vi "WriteForceIni1#.vi"(1 "configuration file path":path=path "E:/LabVIEW/福尔达/AppData") -> ()   [LabVIEW 2018]
uses:
  <vilib>/Utility/config.llb/Write Key (Double).vi
  <vilib>/Utility/config.llb/NI_LVConfig.lvlib
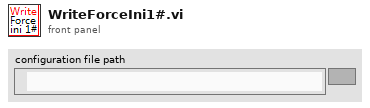
[diagram p1: front panel]
types:
  T1 = typedef "NI_LVConfig.lvlib/Config Data RefNum.ctl" = refnum<k1>
  T2 = cluster{"选择":enum16{"Fx", "Fy", "Fz", "Mx", "My", "Mz"}, "系数x":sgl, "系数+":sgl, "上限":sgl, "下限":sgl, "Ymax":dbl, "Ymin":dbl, "点数":dbl, "锁系数x":sgl, "锁上限":sgl, "锁下限":sgl, "锁系数+":sgl, "起点":dbl, "终点":dbl, "锁起点":dbl, "锁终点":dbl, "上参考":sgl, "下参考":sgl, "基准":sgl}
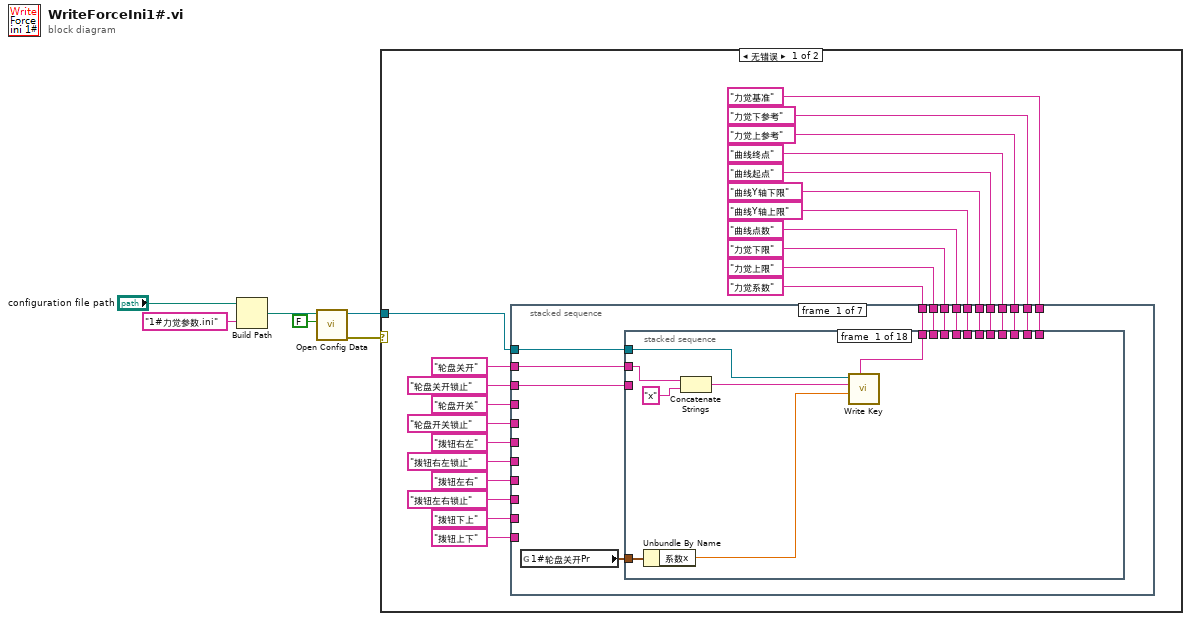
[diagram p0: block diagram]
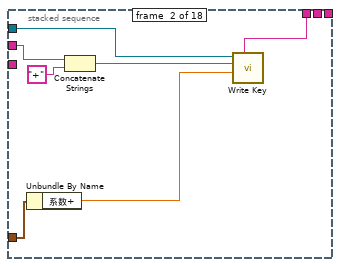
[diagram p2: hidden frame]
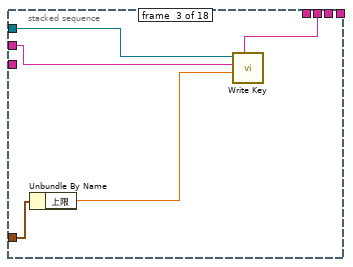
[diagram p3: hidden frame]
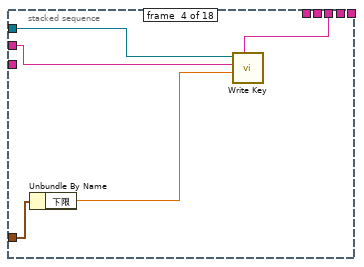
[diagram p4: hidden frame]
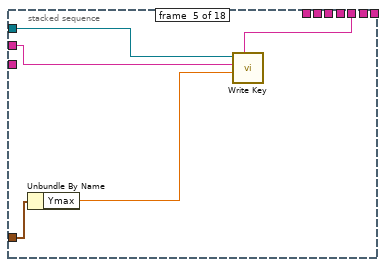
[diagram p5: hidden frame]
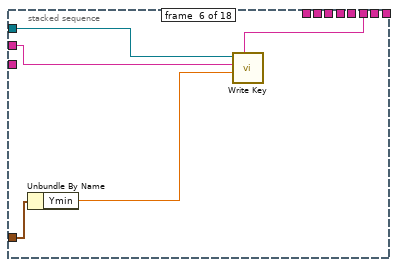
[diagram p6: hidden frame]
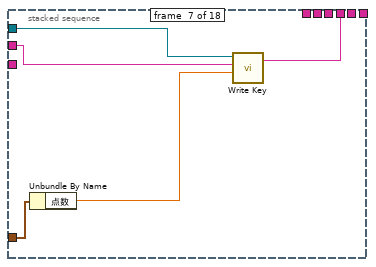
[diagram p7: hidden frame]
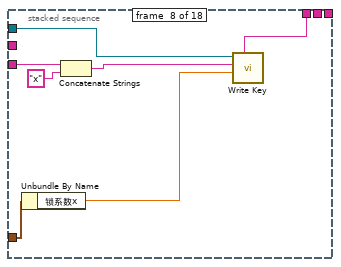
[diagram p8: hidden frame]
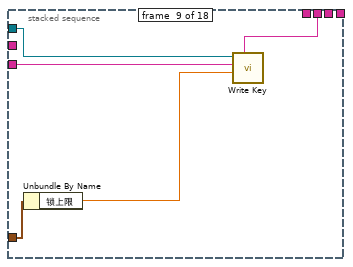
[diagram p9: hidden frame]
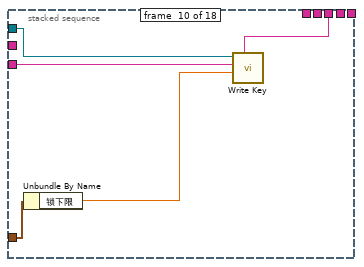
[diagram p10: hidden frame]
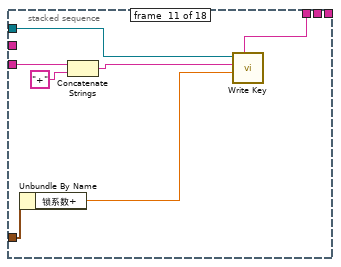
[diagram p11: hidden frame]
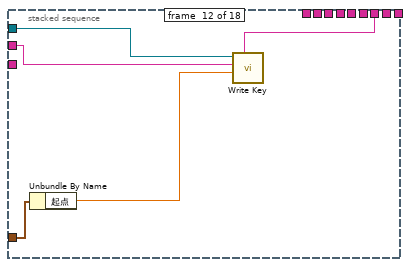
[diagram p12: hidden frame]
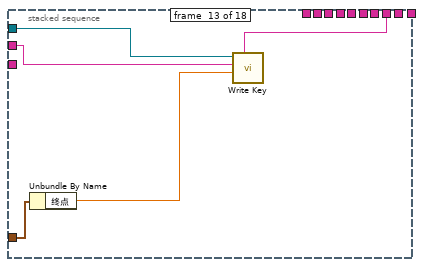
[diagram p13: hidden frame]
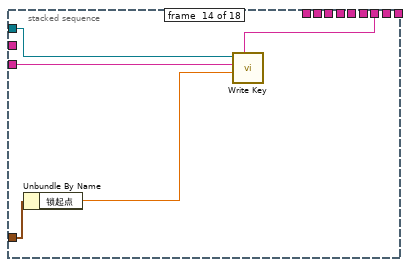
[diagram p14: hidden frame]
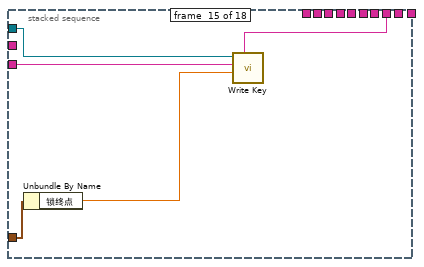
[diagram p15: hidden frame]
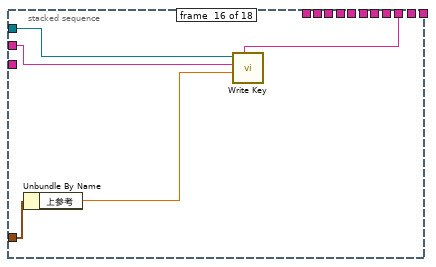
[diagram p16: hidden frame]
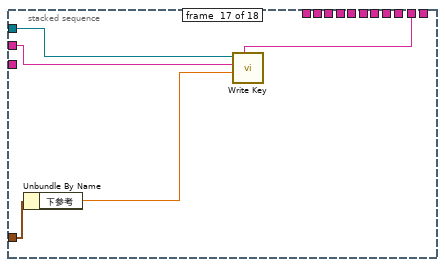
[diagram p17: hidden frame]
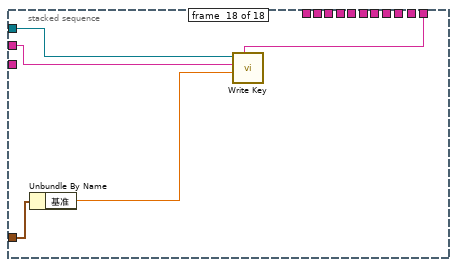
[diagram p18: hidden frame]
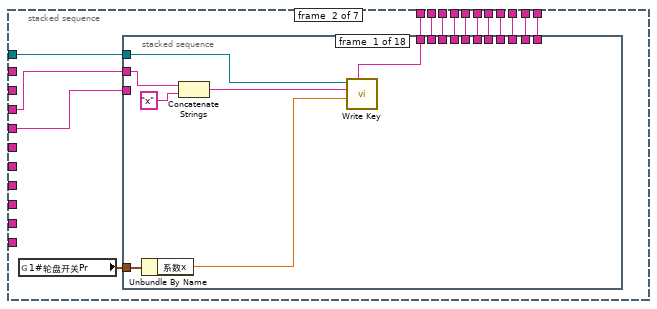
[diagram p19: hidden frame]
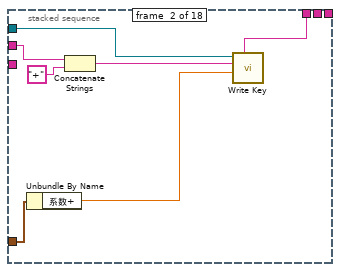
[diagram p20: hidden frame]
diagram:
  n1 = Build Path(base path="configuration file path", name or relative path="1#力觉参数.ini" ("名称或相对路径")) -> (appended path=w6:path)
  n2 = call <vilib>:"Open Config Data.vi"("create file if necessary (T)"=FALSE, "configuration file path"=w6) -> ("error out"=w1:errorcluster, "refnum"=w4:T1)  [unwired: 7 in, 1 out]
  n3 = case shown="无错误" w1 {
    tunnel: w4 -> [w12 w639]
    frame No Error {
      n4 = stacked-sequence {
        tunnel: w12 -> [w32 w147 w260 w373 w485 w563 w637]
        tunnel: "轮盘关开" -> [w42 _ _ _ _ _ _]
        tunnel: "拨钮上下" -> [_ _ _ _ _ w559 _]
        tunnel: "拨钮下上" -> [_ _ _ _ w481 _ _]
        tunnel: "拨钮左右" -> [_ _ _ w369 _ _ _]
        tunnel: "拨钮右左" -> [_ _ w256 _ _ _ _]
        tunnel: "轮盘开关锁止" -> [_ w142 _ _ _ _ _]
        tunnel: "轮盘开关" -> [_ w143 _ _ _ _ _]
        tunnel: "轮盘关开锁止" -> [w33 _ _ _ _ _ _]
        tunnel: "力觉系数" -> [w41 w155 w268 w381 w493 w571 _]
        tunnel: "力觉上限" -> [w40 w154 w267 w380 w492 w570 _]
        tunnel: "力觉下限" -> [w39 w153 w266 w379 w491 w569 _]
        tunnel: "曲线点数" -> [w38 w152 w265 w378 w490 w568 _]
        tunnel: "曲线Y轴上限" -> [w37 w151 w264 w377 w489 w567 _]
        tunnel: "曲线Y轴下限" -> [w36 w150 w263 w376 w488 w566 _]
        tunnel: "曲线起点" -> [w35 w149 w262 w375 w487 w565 _]
        tunnel: "曲线终点" -> [w34 w148 w261 w374 w486 w564 _]
        tunnel: "力觉上参考" -> [w31 w146 w259 w372 w484 w562 _]
        tunnel: "力觉下参考" -> [w30 w145 w258 w371 w483 w561 _]
        tunnel: "力觉基准" -> [w29 w144 w257 w370 w482 w560 _]
        tunnel: "拨钮右左锁止" -> [_ _ w255 _ _ _ _]
        tunnel: "拨钮左右锁止" -> [_ _ _ w368 _ _ _]
        frame #0 {
          n5 = global read "全局F参数.vi" "1#轮盘关开Pr"() -> (w43:T2)
          n6 = stacked-sequence {
            tunnel: w42 -> [w44 w51 w59 w64 w69 w74 w79 _ _ _ _ w108 w113 _ _ w127 w132 w137]
            tunnel: w43 -> [w50 w57 w62 w67 w72 w77 w82 w89 w94 w99 w106 w111 w116 w121 w126 w131 w136 w141]
            tunnel: w32 -> [w48 w55 w60 w65 w70 w75 w80 w87 w92 w97 w104 w109 w114 w119 w124 w129 w134 w139]
            tunnel: w41 -> [w47 w54 _ _ _ _ _ w86 _ _ w100 _ _ _ _ _ _ _]
            tunnel: w40 -> [_ _ w58 _ _ _ _ _ w90 _ _ _ _ _ _ _ _ _]
            tunnel: w39 -> [_ _ _ w63 _ _ _ _ _ w95 _ _ _ _ _ _ _ _]
            tunnel: w38 -> [_ _ _ _ _ _ w78 _ _ _ _ _ _ _ _ _ _ _]
            tunnel: w37 -> [_ _ _ _ w68 _ _ _ _ _ _ _ _ _ _ _ _ _]
            tunnel: w36 -> [_ _ _ _ _ w73 _ _ _ _ _ _ _ _ _ _ _ _]
            tunnel: w35 -> [_ _ _ _ _ _ _ _ _ _ _ w107 _ w117 _ _ _ _]
            tunnel: w34 -> [_ _ _ _ _ _ _ _ _ _ _ _ w112 _ w122 _ _ _]
            tunnel: w33 -> [_ _ _ _ _ _ _ w85 w91 w96 w103 _ _ w118 w123 _ _ _]
            tunnel: w31 -> [_ _ _ _ _ _ _ _ _ _ _ _ _ _ _ w128 _ _]
            tunnel: w30 -> [_ _ _ _ _ _ _ _ _ _ _ _ _ _ _ _ w133 _]
            tunnel: w29 -> [_ _ _ _ _ _ _ _ _ _ _ _ _ _ _ _ _ w138]
            frame #0 {
              n7 = Unbundle By Name(w50) -> ("系数x"=w49:sgl)
              n8 = Concatenate Strings(w44, "x") -> (w45:string)
              n9 = call-poly <vilib>:"Write Key.vi"("section"=w47, "value"=w49, "key"=w45, "refnum"=w48) -> ()  [unwired: 5 in, 3 out]
            }
            frame #1 {
              n10 = Unbundle By Name(w57) -> ("系数+"=w56:sgl)
              n11 = Concatenate Strings(w51, "+") -> (w52:string)
              n12 = call-poly <vilib>:"Write Key.vi"("section"=w54, "value"=w56, "key"=w52, "refnum"=w55) -> ()  [unwired: 5 in, 3 out]
            }
            frame #2 {
              n13 = Unbundle By Name(w62) -> ("上限"=w61:sgl)
              n14 = call-poly <vilib>:"Write Key.vi"("section"=w58, "value"=w61, "key"=w59, "refnum"=w60) -> ()  [unwired: 5 in, 3 out]
            }
            frame #3 {
              n15 = Unbundle By Name(w67) -> ("下限"=w66:sgl)
              n16 = call-poly <vilib>:"Write Key.vi"("section"=w63, "value"=w66, "key"=w64, "refnum"=w65) -> ()  [unwired: 5 in, 3 out]
            }
            frame #4 {
              n17 = Unbundle By Name(w72) -> ("Ymax"=w71:dbl)
              n18 = call-poly <vilib>:"Write Key.vi"("section"=w68, "value"=w71, "key"=w69, "refnum"=w70) -> ()  [unwired: 5 in, 3 out]
            }
            frame #5 {
              n19 = Unbundle By Name(w77) -> ("Ymin"=w76:dbl)
              n20 = call-poly <vilib>:"Write Key.vi"("section"=w73, "value"=w76, "key"=w74, "refnum"=w75) -> ()  [unwired: 5 in, 3 out]
            }
            frame #6 {
              n21 = Unbundle By Name(w82) -> ("点数"=w81:dbl)
              n22 = call-poly <vilib>:"Write Key.vi"("section"=w78, "value"=w81, "key"=w79, "refnum"=w80) -> ()  [unwired: 5 in, 3 out]
            }
            frame #7 {
              n23 = Unbundle By Name(w89) -> ("锁系数x"=w88:sgl)
              n24 = Concatenate Strings(w85, "x") -> (w84:string)
              n25 = call-poly <vilib>:"Write Key.vi"("section"=w86, "value"=w88, "key"=w84, "refnum"=w87) -> ()  [unwired: 5 in, 3 out]
            }
            frame #8 {
              n26 = Unbundle By Name(w94) -> ("锁上限"=w93:sgl)
              n27 = call-poly <vilib>:"Write Key.vi"("section"=w90, "value"=w93, "key"=w91, "refnum"=w92) -> ()  [unwired: 5 in, 3 out]
            }
            frame #9 {
              n28 = Unbundle By Name(w99) -> ("锁下限"=w98:sgl)
              n29 = call-poly <vilib>:"Write Key.vi"("section"=w95, "value"=w98, "key"=w96, "refnum"=w97) -> ()  [unwired: 5 in, 3 out]
            }
            frame #10 {
              n30 = Unbundle By Name(w106) -> ("锁系数+"=w105:sgl)
              n31 = Concatenate Strings(w103, "+") -> (w102:string)
              n32 = call-poly <vilib>:"Write Key.vi"("section"=w100, "value"=w105, "key"=w102, "refnum"=w104) -> ()  [unwired: 5 in, 3 out]
            }
            frame #11 {
              n33 = Unbundle By Name(w111) -> ("起点"=w110:dbl)
              n34 = call-poly <vilib>:"Write Key.vi"("section"=w107, "value"=w110, "key"=w108, "refnum"=w109) -> ()  [unwired: 5 in, 3 out]
            }
            frame #12 {
              n35 = Unbundle By Name(w116) -> ("终点"=w115:dbl)
              n36 = call-poly <vilib>:"Write Key.vi"("section"=w112, "value"=w115, "key"=w113, "refnum"=w114) -> ()  [unwired: 5 in, 3 out]
            }
            frame #13 {
              n37 = Unbundle By Name(w121) -> ("锁起点"=w120:dbl)
              n38 = call-poly <vilib>:"Write Key.vi"("section"=w117, "value"=w120, "key"=w118, "refnum"=w119) -> ()  [unwired: 5 in, 3 out]
            }
            frame #14 {
              n39 = Unbundle By Name(w126) -> ("锁终点"=w125:dbl)
              n40 = call-poly <vilib>:"Write Key.vi"("section"=w122, "value"=w125, "key"=w123, "refnum"=w124) -> ()  [unwired: 5 in, 3 out]
            }
            frame #15 {
              n41 = Unbundle By Name(w131) -> ("上参考"=w130:sgl)
              n42 = call-poly <vilib>:"Write Key.vi"("section"=w128, "value"=w130, "key"=w127, "refnum"=w129) -> ()  [unwired: 5 in, 3 out]
            }
            frame #16 {
              n43 = Unbundle By Name(w136) -> ("下参考"=w135:sgl)
              n44 = call-poly <vilib>:"Write Key.vi"("section"=w133, "value"=w135, "key"=w132, "refnum"=w134) -> ()  [unwired: 5 in, 3 out]
            }
            frame #17 {
              n45 = Unbundle By Name(w141) -> ("基准"=w140:sgl)
              n46 = call-poly <vilib>:"Write Key.vi"("section"=w138, "value"=w140, "key"=w137, "refnum"=w139) -> ()  [unwired: 5 in, 3 out]
            }
          }
        }
        frame #1 {
          n47 = global read "全局F参数.vi" "1#轮盘开关Pr"() -> (w156:T2)
          n48 = stacked-sequence {
            tunnel: w143 -> [w157 w164 w172 w177 w182 w187 w192 _ _ _ _ w221 w226 _ _ w240 w245 w250]
            tunnel: w156 -> [w163 w170 w175 w180 w185 w190 w195 w202 w207 w212 w219 w224 w229 w234 w239 w244 w249 w254]
            tunnel: w147 -> [w161 w168 w173 w178 w183 w188 w193 w200 w205 w210 w217 w222 w227 w232 w237 w242 w247 w252]
            tunnel: w155 -> [w160 w167 _ _ _ _ _ w199 _ _ w213 _ _ _ _ _ _ _]
            tunnel: w154 -> [_ _ w171 _ _ _ _ _ w203 _ _ _ _ _ _ _ _ _]
            tunnel: w153 -> [_ _ _ w176 _ _ _ _ _ w208 _ _ _ _ _ _ _ _]
            tunnel: w152 -> [_ _ _ _ _ _ w191 _ _ _ _ _ _ _ _ _ _ _]
            tunnel: w151 -> [_ _ _ _ w181 _ _ _ _ _ _ _ _ _ _ _ _ _]
            tunnel: w150 -> [_ _ _ _ _ w186 _ _ _ _ _ _ _ _ _ _ _ _]
            tunnel: w149 -> [_ _ _ _ _ _ _ _ _ _ _ w220 _ w230 _ _ _ _]
            tunnel: w148 -> [_ _ _ _ _ _ _ _ _ _ _ _ w225 _ w235 _ _ _]
            tunnel: w142 -> [_ _ _ _ _ _ _ w198 w204 w209 w216 _ _ w231 w236 _ _ _]
            tunnel: w146 -> [_ _ _ _ _ _ _ _ _ _ _ _ _ _ _ w241 _ _]
            tunnel: w145 -> [_ _ _ _ _ _ _ _ _ _ _ _ _ _ _ _ w246 _]
            tunnel: w144 -> [_ _ _ _ _ _ _ _ _ _ _ _ _ _ _ _ _ w251]
            frame #0 {
              n49 = Unbundle By Name(w163) -> ("系数x"=w162:sgl)
              n50 = Concatenate Strings(w157, "x") -> (w158:string)
              n51 = call-poly <vilib>:"Write Key.vi"("section"=w160, "value"=w162, "key"=w158, "refnum"=w161) -> ()  [unwired: 5 in, 3 out]
            }
            frame #1 {
              n52 = Unbundle By Name(w170) -> ("系数+"=w169:sgl)
              n53 = Concatenate Strings(w164, "+") -> (w165:string)
              n54 = call-poly <vilib>:"Write Key.vi"("section"=w167, "value"=w169, "key"=w165, "refnum"=w168) -> ()  [unwired: 5 in, 3 out]
            }
            frame #2 {
              n55 = Unbundle By Name(w175) -> ("上限"=w174:sgl)
              n56 = call-poly <vilib>:"Write Key.vi"("section"=w171, "value"=w174, "key"=w172, "refnum"=w173) -> ()  [unwired: 5 in, 3 out]
            }
            frame #3 {
              n57 = Unbundle By Name(w180) -> ("下限"=w179:sgl)
              n58 = call-poly <vilib>:"Write Key.vi"("section"=w176, "value"=w179, "key"=w177, "refnum"=w178) -> ()  [unwired: 5 in, 3 out]
            }
            frame #4 {
              n59 = Unbundle By Name(w185) -> ("Ymax"=w184:dbl)
              n60 = call-poly <vilib>:"Write Key.vi"("section"=w181, "value"=w184, "key"=w182, "refnum"=w183) -> ()  [unwired: 5 in, 3 out]
            }
            frame #5 {
              n61 = Unbundle By Name(w190) -> ("Ymin"=w189:dbl)
              n62 = call-poly <vilib>:"Write Key.vi"("section"=w186, "value"=w189, "key"=w187, "refnum"=w188) -> ()  [unwired: 5 in, 3 out]
            }
            frame #6 {
              n63 = Unbundle By Name(w195) -> ("点数"=w194:dbl)
              n64 = call-poly <vilib>:"Write Key.vi"("section"=w191, "value"=w194, "key"=w192, "refnum"=w193) -> ()  [unwired: 5 in, 3 out]
            }
            frame #7 {
              n65 = Unbundle By Name(w202) -> ("锁系数x"=w201:sgl)
              n66 = Concatenate Strings(w198, "x") -> (w197:string)
              n67 = call-poly <vilib>:"Write Key.vi"("section"=w199, "value"=w201, "key"=w197, "refnum"=w200) -> ()  [unwired: 5 in, 3 out]
            }
            frame #8 {
              n68 = Unbundle By Name(w207) -> ("锁上限"=w206:sgl)
              n69 = call-poly <vilib>:"Write Key.vi"("section"=w203, "value"=w206, "key"=w204, "refnum"=w205) -> ()  [unwired: 5 in, 3 out]
            }
            frame #9 {
              n70 = Unbundle By Name(w212) -> ("锁下限"=w211:sgl)
              n71 = call-poly <vilib>:"Write Key.vi"("section"=w208, "value"=w211, "key"=w209, "refnum"=w210) -> ()  [unwired: 5 in, 3 out]
            }
            frame #10 {
              n72 = Unbundle By Name(w219) -> ("锁系数+"=w218:sgl)
              n73 = Concatenate Strings(w216, "+") -> (w215:string)
              n74 = call-poly <vilib>:"Write Key.vi"("section"=w213, "value"=w218, "key"=w215, "refnum"=w217) -> ()  [unwired: 5 in, 3 out]
            }
            frame #11 {
              n75 = Unbundle By Name(w224) -> ("起点"=w223:dbl)
              n76 = call-poly <vilib>:"Write Key.vi"("section"=w220, "value"=w223, "key"=w221, "refnum"=w222) -> ()  [unwired: 5 in, 3 out]
            }
            frame #12 {
              n77 = Unbundle By Name(w229) -> ("终点"=w228:dbl)
              n78 = call-poly <vilib>:"Write Key.vi"("section"=w225, "value"=w228, "key"=w226, "refnum"=w227) -> ()  [unwired: 5 in, 3 out]
            }
            frame #13 {
              n79 = Unbundle By Name(w234) -> ("锁起点"=w233:dbl)
              n80 = call-poly <vilib>:"Write Key.vi"("section"=w230, "value"=w233, "key"=w231, "refnum"=w232) -> ()  [unwired: 5 in, 3 out]
            }
            frame #14 {
              n81 = Unbundle By Name(w239) -> ("锁终点"=w238:dbl)
              n82 = call-poly <vilib>:"Write Key.vi"("section"=w235, "value"=w238, "key"=w236, "refnum"=w237) -> ()  [unwired: 5 in, 3 out]
            }
            frame #15 {
              n83 = Unbundle By Name(w244) -> ("上参考"=w243:sgl)
              n84 = call-poly <vilib>:"Write Key.vi"("section"=w241, "value"=w243, "key"=w240, "refnum"=w242) -> ()  [unwired: 5 in, 3 out]
            }
            frame #16 {
              n85 = Unbundle By Name(w249) -> ("下参考"=w248:sgl)
              n86 = call-poly <vilib>:"Write Key.vi"("section"=w246, "value"=w248, "key"=w245, "refnum"=w247) -> ()  [unwired: 5 in, 3 out]
            }
            frame #17 {
              n87 = Unbundle By Name(w254) -> ("基准"=w253:sgl)
              n88 = call-poly <vilib>:"Write Key.vi"("section"=w251, "value"=w253, "key"=w250, "refnum"=w252) -> ()  [unwired: 5 in, 3 out]
            }
          }
        }
        frame #2 {
          n89 = global read "全局F参数.vi" "1#拨钮右左Pr"() -> (w269:T2)
          n90 = stacked-sequence {
            tunnel: w256 -> [w270 w277 w285 w290 w295 w300 w305 _ _ _ _ w334 w339 _ _ w353 w358 w363]
            tunnel: w269 -> [w276 w283 w288 w293 w298 w303 w308 w315 w320 w325 w332 w337 w342 w347 w352 w357 w362 w367]
            tunnel: w260 -> [w274 w281 w286 w291 w296 w301 w306 w313 w318 w323 w330 w335 w340 w345 w350 w355 w360 w365]
            tunnel: w268 -> [w273 w280 _ _ _ _ _ w312 _ _ w326 _ _ _ _ _ _ _]
            tunnel: w267 -> [_ _ w284 _ _ _ _ _ w316 _ _ _ _ _ _ _ _ _]
            tunnel: w266 -> [_ _ _ w289 _ _ _ _ _ w321 _ _ _ _ _ _ _ _]
            tunnel: w265 -> [_ _ _ _ _ _ w304 _ _ _ _ _ _ _ _ _ _ _]
            tunnel: w264 -> [_ _ _ _ w294 _ _ _ _ _ _ _ _ _ _ _ _ _]
            tunnel: w263 -> [_ _ _ _ _ w299 _ _ _ _ _ _ _ _ _ _ _ _]
            tunnel: w262 -> [_ _ _ _ _ _ _ _ _ _ _ w333 _ w343 _ _ _ _]
            tunnel: w261 -> [_ _ _ _ _ _ _ _ _ _ _ _ w338 _ w348 _ _ _]
            tunnel: w255 -> [_ _ _ _ _ _ _ w311 w317 w322 w329 _ _ w344 w349 _ _ _]
            tunnel: w259 -> [_ _ _ _ _ _ _ _ _ _ _ _ _ _ _ w354 _ _]
            tunnel: w258 -> [_ _ _ _ _ _ _ _ _ _ _ _ _ _ _ _ w359 _]
            tunnel: w257 -> [_ _ _ _ _ _ _ _ _ _ _ _ _ _ _ _ _ w364]
            frame #0 {
              n91 = Unbundle By Name(w276) -> ("系数x"=w275:sgl)
              n92 = Concatenate Strings(w270, "x") -> (w271:string)
              n93 = call-poly <vilib>:"Write Key.vi"("section"=w273, "value"=w275, "key"=w271, "refnum"=w274) -> ()  [unwired: 5 in, 3 out]
            }
            frame #1 {
              n94 = Unbundle By Name(w283) -> ("系数+"=w282:sgl)
              n95 = Concatenate Strings(w277, "+") -> (w278:string)
              n96 = call-poly <vilib>:"Write Key.vi"("section"=w280, "value"=w282, "key"=w278, "refnum"=w281) -> ()  [unwired: 5 in, 3 out]
            }
            frame #2 {
              n97 = Unbundle By Name(w288) -> ("上限"=w287:sgl)
              n98 = call-poly <vilib>:"Write Key.vi"("section"=w284, "value"=w287, "key"=w285, "refnum"=w286) -> ()  [unwired: 5 in, 3 out]
            }
            frame #3 {
              n99 = Unbundle By Name(w293) -> ("下限"=w292:sgl)
              n100 = call-poly <vilib>:"Write Key.vi"("section"=w289, "value"=w292, "key"=w290, "refnum"=w291) -> ()  [unwired: 5 in, 3 out]
            }
            frame #4 {
              n101 = Unbundle By Name(w298) -> ("Ymax"=w297:dbl)
              n102 = call-poly <vilib>:"Write Key.vi"("section"=w294, "value"=w297, "key"=w295, "refnum"=w296) -> ()  [unwired: 5 in, 3 out]
            }
            frame #5 {
              n103 = Unbundle By Name(w303) -> ("Ymin"=w302:dbl)
              n104 = call-poly <vilib>:"Write Key.vi"("section"=w299, "value"=w302, "key"=w300, "refnum"=w301) -> ()  [unwired: 5 in, 3 out]
            }
            frame #6 {
              n105 = Unbundle By Name(w308) -> ("点数"=w307:dbl)
              n106 = call-poly <vilib>:"Write Key.vi"("section"=w304, "value"=w307, "key"=w305, "refnum"=w306) -> ()  [unwired: 5 in, 3 out]
            }
            frame #7 {
              n107 = Unbundle By Name(w315) -> ("锁系数x"=w314:sgl)
              n108 = Concatenate Strings(w311, "x") -> (w310:string)
              n109 = call-poly <vilib>:"Write Key.vi"("section"=w312, "value"=w314, "key"=w310, "refnum"=w313) -> ()  [unwired: 5 in, 3 out]
            }
            frame #8 {
              n110 = Unbundle By Name(w320) -> ("锁上限"=w319:sgl)
              n111 = call-poly <vilib>:"Write Key.vi"("section"=w316, "value"=w319, "key"=w317, "refnum"=w318) -> ()  [unwired: 5 in, 3 out]
            }
            frame #9 {
              n112 = Unbundle By Name(w325) -> ("锁下限"=w324:sgl)
              n113 = call-poly <vilib>:"Write Key.vi"("section"=w321, "value"=w324, "key"=w322, "refnum"=w323) -> ()  [unwired: 5 in, 3 out]
            }
            frame #10 {
              n114 = Unbundle By Name(w332) -> ("锁系数+"=w331:sgl)
              n115 = Concatenate Strings(w329, "+") -> (w328:string)
              n116 = call-poly <vilib>:"Write Key.vi"("section"=w326, "value"=w331, "key"=w328, "refnum"=w330) -> ()  [unwired: 5 in, 3 out]
            }
            frame #11 {
              n117 = Unbundle By Name(w337) -> ("起点"=w336:dbl)
              n118 = call-poly <vilib>:"Write Key.vi"("section"=w333, "value"=w336, "key"=w334, "refnum"=w335) -> ()  [unwired: 5 in, 3 out]
            }
            frame #12 {
              n119 = Unbundle By Name(w342) -> ("终点"=w341:dbl)
              n120 = call-poly <vilib>:"Write Key.vi"("section"=w338, "value"=w341, "key"=w339, "refnum"=w340) -> ()  [unwired: 5 in, 3 out]
            }
            frame #13 {
              n121 = Unbundle By Name(w347) -> ("锁起点"=w346:dbl)
              n122 = call-poly <vilib>:"Write Key.vi"("section"=w343, "value"=w346, "key"=w344, "refnum"=w345) -> ()  [unwired: 5 in, 3 out]
            }
            frame #14 {
              n123 = Unbundle By Name(w352) -> ("锁终点"=w351:dbl)
              n124 = call-poly <vilib>:"Write Key.vi"("section"=w348, "value"=w351, "key"=w349, "refnum"=w350) -> ()  [unwired: 5 in, 3 out]
            }
            frame #15 {
              n125 = Unbundle By Name(w357) -> ("上参考"=w356:sgl)
              n126 = call-poly <vilib>:"Write Key.vi"("section"=w354, "value"=w356, "key"=w353, "refnum"=w355) -> ()  [unwired: 5 in, 3 out]
            }
            frame #16 {
              n127 = Unbundle By Name(w362) -> ("下参考"=w361:sgl)
              n128 = call-poly <vilib>:"Write Key.vi"("section"=w359, "value"=w361, "key"=w358, "refnum"=w360) -> ()  [unwired: 5 in, 3 out]
            }
            frame #17 {
              n129 = Unbundle By Name(w367) -> ("基准"=w366:sgl)
              n130 = call-poly <vilib>:"Write Key.vi"("section"=w364, "value"=w366, "key"=w363, "refnum"=w365) -> ()  [unwired: 5 in, 3 out]
            }
          }
        }
        frame #3 {
          n131 = global read "全局F参数.vi" "1#拨钮左右Pr"() -> (w382:T2)
          n132 = stacked-sequence {
            tunnel: w369 -> [w383 w390 w398 w403 w408 w413 w418 _ _ _ _ w447 w452 _ _ w466 w471 w476]
            tunnel: w382 -> [w389 w396 w401 w406 w411 w416 w421 w428 w433 w438 w445 w450 w455 w460 w465 w470 w475 w480]
            tunnel: w373 -> [w387 w394 w399 w404 w409 w414 w419 w426 w431 w436 w443 w448 w453 w458 w463 w468 w473 w478]
            tunnel: w381 -> [w386 w393 _ _ _ _ _ w425 _ _ w439 _ _ _ _ _ _ _]
            tunnel: w380 -> [_ _ w397 _ _ _ _ _ w429 _ _ _ _ _ _ _ _ _]
            tunnel: w379 -> [_ _ _ w402 _ _ _ _ _ w434 _ _ _ _ _ _ _ _]
            tunnel: w378 -> [_ _ _ _ _ _ w417 _ _ _ _ _ _ _ _ _ _ _]
            tunnel: w377 -> [_ _ _ _ w407 _ _ _ _ _ _ _ _ _ _ _ _ _]
            tunnel: w376 -> [_ _ _ _ _ w412 _ _ _ _ _ _ _ _ _ _ _ _]
            tunnel: w375 -> [_ _ _ _ _ _ _ _ _ _ _ w446 _ w456 _ _ _ _]
            tunnel: w374 -> [_ _ _ _ _ _ _ _ _ _ _ _ w451 _ w461 _ _ _]
            tunnel: w368 -> [_ _ _ _ _ _ _ w424 w430 w435 w442 _ _ w457 w462 _ _ _]
            tunnel: w372 -> [_ _ _ _ _ _ _ _ _ _ _ _ _ _ _ w467 _ _]
            tunnel: w371 -> [_ _ _ _ _ _ _ _ _ _ _ _ _ _ _ _ w472 _]
            tunnel: w370 -> [_ _ _ _ _ _ _ _ _ _ _ _ _ _ _ _ _ w477]
            frame #0 {
              n133 = Unbundle By Name(w389) -> ("系数x"=w388:sgl)
              n134 = Concatenate Strings(w383, "x") -> (w384:string)
              n135 = call-poly <vilib>:"Write Key.vi"("section"=w386, "value"=w388, "key"=w384, "refnum"=w387) -> ()  [unwired: 5 in, 3 out]
            }
            frame #1 {
              n136 = Unbundle By Name(w396) -> ("系数+"=w395:sgl)
              n137 = Concatenate Strings(w390, "+") -> (w391:string)
              n138 = call-poly <vilib>:"Write Key.vi"("section"=w393, "value"=w395, "key"=w391, "refnum"=w394) -> ()  [unwired: 5 in, 3 out]
            }
            frame #2 {
              n139 = Unbundle By Name(w401) -> ("上限"=w400:sgl)
              n140 = call-poly <vilib>:"Write Key.vi"("section"=w397, "value"=w400, "key"=w398, "refnum"=w399) -> ()  [unwired: 5 in, 3 out]
            }
            frame #3 {
              n141 = Unbundle By Name(w406) -> ("下限"=w405:sgl)
              n142 = call-poly <vilib>:"Write Key.vi"("section"=w402, "value"=w405, "key"=w403, "refnum"=w404) -> ()  [unwired: 5 in, 3 out]
            }
            frame #4 {
              n143 = Unbundle By Name(w411) -> ("Ymax"=w410:dbl)
              n144 = call-poly <vilib>:"Write Key.vi"("section"=w407, "value"=w410, "key"=w408, "refnum"=w409) -> ()  [unwired: 5 in, 3 out]
            }
            frame #5 {
              n145 = Unbundle By Name(w416) -> ("Ymin"=w415:dbl)
              n146 = call-poly <vilib>:"Write Key.vi"("section"=w412, "value"=w415, "key"=w413, "refnum"=w414) -> ()  [unwired: 5 in, 3 out]
            }
            frame #6 {
              n147 = Unbundle By Name(w421) -> ("点数"=w420:dbl)
              n148 = call-poly <vilib>:"Write Key.vi"("section"=w417, "value"=w420, "key"=w418, "refnum"=w419) -> ()  [unwired: 5 in, 3 out]
            }
            frame #7 {
              n149 = Unbundle By Name(w428) -> ("锁系数x"=w427:sgl)
              n150 = Concatenate Strings(w424, "x") -> (w423:string)
              n151 = call-poly <vilib>:"Write Key.vi"("section"=w425, "value"=w427, "key"=w423, "refnum"=w426) -> ()  [unwired: 5 in, 3 out]
            }
            frame #8 {
              n152 = Unbundle By Name(w433) -> ("锁上限"=w432:sgl)
              n153 = call-poly <vilib>:"Write Key.vi"("section"=w429, "value"=w432, "key"=w430, "refnum"=w431) -> ()  [unwired: 5 in, 3 out]
            }
            frame #9 {
              n154 = Unbundle By Name(w438) -> ("锁下限"=w437:sgl)
              n155 = call-poly <vilib>:"Write Key.vi"("section"=w434, "value"=w437, "key"=w435, "refnum"=w436) -> ()  [unwired: 5 in, 3 out]
            }
            frame #10 {
              n156 = Unbundle By Name(w445) -> ("锁系数+"=w444:sgl)
              n157 = Concatenate Strings(w442, "+") -> (w441:string)
              n158 = call-poly <vilib>:"Write Key.vi"("section"=w439, "value"=w444, "key"=w441, "refnum"=w443) -> ()  [unwired: 5 in, 3 out]
            }
            frame #11 {
              n159 = Unbundle By Name(w450) -> ("起点"=w449:dbl)
              n160 = call-poly <vilib>:"Write Key.vi"("section"=w446, "value"=w449, "key"=w447, "refnum"=w448) -> ()  [unwired: 5 in, 3 out]
            }
            frame #12 {
              n161 = Unbundle By Name(w455) -> ("终点"=w454:dbl)
              n162 = call-poly <vilib>:"Write Key.vi"("section"=w451, "value"=w454, "key"=w452, "refnum"=w453) -> ()  [unwired: 5 in, 3 out]
            }
            frame #13 {
              n163 = Unbundle By Name(w460) -> ("锁起点"=w459:dbl)
              n164 = call-poly <vilib>:"Write Key.vi"("section"=w456, "value"=w459, "key"=w457, "refnum"=w458) -> ()  [unwired: 5 in, 3 out]
            }
            frame #14 {
              n165 = Unbundle By Name(w465) -> ("锁终点"=w464:dbl)
              n166 = call-poly <vilib>:"Write Key.vi"("section"=w461, "value"=w464, "key"=w462, "refnum"=w463) -> ()  [unwired: 5 in, 3 out]
            }
            frame #15 {
              n167 = Unbundle By Name(w470) -> ("上参考"=w469:sgl)
              n168 = call-poly <vilib>:"Write Key.vi"("section"=w467, "value"=w469, "key"=w466, "refnum"=w468) -> ()  [unwired: 5 in, 3 out]
            }
            frame #16 {
              n169 = Unbundle By Name(w475) -> ("下参考"=w474:sgl)
              n170 = call-poly <vilib>:"Write Key.vi"("section"=w472, "value"=w474, "key"=w471, "refnum"=w473) -> ()  [unwired: 5 in, 3 out]
            }
            frame #17 {
              n171 = Unbundle By Name(w480) -> ("基准"=w479:sgl)
              n172 = call-poly <vilib>:"Write Key.vi"("section"=w477, "value"=w479, "key"=w476, "refnum"=w478) -> ()  [unwired: 5 in, 3 out]
            }
          }
        }
        frame #4 {
          n173 = global read "全局F参数.vi" "1#拨钮下上Pr"() -> (w494:T2)
          n174 = stacked-sequence {
            tunnel: w481 -> [w496 w503 w510 w515 w520 w525 w530 w535 w540 w545 w550 w555]
            tunnel: w494 -> [w501 w508 w513 w518 w523 w528 w533 w538 w543 w548 w553 w558]
            tunnel: w485 -> [w499 w506 w511 w516 w521 w526 w531 w536 w541 w546 w551 w556]
            tunnel: w493 -> [w498 w505 _ _ _ _ _ _ _ _ _ _]
            tunnel: w492 -> [_ _ w509 _ _ _ _ _ _ _ _ _]
            tunnel: w491 -> [_ _ _ w514 _ _ _ _ _ _ _ _]
            tunnel: w490 -> [_ _ _ _ _ _ w529 _ _ _ _ _]
            tunnel: w489 -> [_ _ _ _ w519 _ _ _ _ _ _ _]
            tunnel: w488 -> [_ _ _ _ _ w524 _ _ _ _ _ _]
            tunnel: w487 -> [_ _ _ _ _ _ _ w534 _ _ _ _]
            tunnel: w486 -> [_ _ _ _ _ _ _ _ w539 _ _ _]
            tunnel: w484 -> [_ _ _ _ _ _ _ _ _ w544 _ _]
            tunnel: w483 -> [_ _ _ _ _ _ _ _ _ _ w549 _]
            tunnel: w482 -> [_ _ _ _ _ _ _ _ _ _ _ w554]
            frame #0 {
              n175 = Unbundle By Name(w501) -> ("系数x"=w500:sgl)
              n176 = Concatenate Strings(w496, "x") -> (w495:string)
              n177 = call-poly <vilib>:"Write Key.vi"("section"=w498, "value"=w500, "key"=w495, "refnum"=w499) -> ()  [unwired: 5 in, 3 out]
            }
            frame #1 {
              n178 = Unbundle By Name(w508) -> ("系数+"=w507:sgl)
              n179 = Concatenate Strings(w503, "+") -> (w502:string)
              n180 = call-poly <vilib>:"Write Key.vi"("section"=w505, "value"=w507, "key"=w502, "refnum"=w506) -> ()  [unwired: 5 in, 3 out]
            }
            frame #2 {
              n181 = Unbundle By Name(w513) -> ("上限"=w512:sgl)
              n182 = call-poly <vilib>:"Write Key.vi"("section"=w509, "value"=w512, "key"=w510, "refnum"=w511) -> ()  [unwired: 5 in, 3 out]
            }
            frame #3 {
              n183 = Unbundle By Name(w518) -> ("下限"=w517:sgl)
              n184 = call-poly <vilib>:"Write Key.vi"("section"=w514, "value"=w517, "key"=w515, "refnum"=w516) -> ()  [unwired: 5 in, 3 out]
            }
            frame #4 {
              n185 = Unbundle By Name(w523) -> ("Ymax"=w522:dbl)
              n186 = call-poly <vilib>:"Write Key.vi"("section"=w519, "value"=w522, "key"=w520, "refnum"=w521) -> ()  [unwired: 5 in, 3 out]
            }
            frame #5 {
              n187 = Unbundle By Name(w528) -> ("Ymin"=w527:dbl)
              n188 = call-poly <vilib>:"Write Key.vi"("section"=w524, "value"=w527, "key"=w525, "refnum"=w526) -> ()  [unwired: 5 in, 3 out]
            }
            frame #6 {
              n189 = Unbundle By Name(w533) -> ("点数"=w532:dbl)
              n190 = call-poly <vilib>:"Write Key.vi"("section"=w529, "value"=w532, "key"=w530, "refnum"=w531) -> ()  [unwired: 5 in, 3 out]
            }
            frame #7 {
              n191 = Unbundle By Name(w538) -> ("起点"=w537:dbl)
              n192 = call-poly <vilib>:"Write Key.vi"("section"=w534, "value"=w537, "key"=w535, "refnum"=w536) -> ()  [unwired: 5 in, 3 out]
            }
            frame #8 {
              n193 = Unbundle By Name(w543) -> ("终点"=w542:dbl)
              n194 = call-poly <vilib>:"Write Key.vi"("section"=w539, "value"=w542, "key"=w540, "refnum"=w541) -> ()  [unwired: 5 in, 3 out]
            }
            frame #9 {
              n195 = Unbundle By Name(w548) -> ("上参考"=w547:sgl)
              n196 = call-poly <vilib>:"Write Key.vi"("section"=w544, "value"=w547, "key"=w545, "refnum"=w546) -> ()  [unwired: 5 in, 3 out]
            }
            frame #10 {
              n197 = Unbundle By Name(w553) -> ("下参考"=w552:sgl)
              n198 = call-poly <vilib>:"Write Key.vi"("section"=w549, "value"=w552, "key"=w550, "refnum"=w551) -> ()  [unwired: 5 in, 3 out]
            }
            frame #11 {
              n199 = Unbundle By Name(w558) -> ("基准"=w557:sgl)
              n200 = call-poly <vilib>:"Write Key.vi"("section"=w554, "value"=w557, "key"=w555, "refnum"=w556) -> ()  [unwired: 5 in, 3 out]
            }
          }
        }
        frame #5 {
          n201 = global read "全局F参数.vi" "1#拨钮上下Pr"() -> (w572:T2)
          n202 = stacked-sequence {
            tunnel: w559 -> [w574 w581 w588 w593 w598 w603 w608 w613 w618 w623 w628 w633]
            tunnel: w572 -> [w579 w586 w591 w596 w601 w606 w611 w616 w621 w626 w631 w636]
            tunnel: w563 -> [w577 w584 w589 w594 w599 w604 w609 w614 w619 w624 w629 w634]
            tunnel: w571 -> [w576 w583 _ _ _ _ _ _ _ _ _ _]
            tunnel: w570 -> [_ _ w587 _ _ _ _ _ _ _ _ _]
            tunnel: w569 -> [_ _ _ w592 _ _ _ _ _ _ _ _]
            tunnel: w568 -> [_ _ _ _ _ _ w607 _ _ _ _ _]
            tunnel: w567 -> [_ _ _ _ w597 _ _ _ _ _ _ _]
            tunnel: w566 -> [_ _ _ _ _ w602 _ _ _ _ _ _]
            tunnel: w565 -> [_ _ _ _ _ _ _ w612 _ _ _ _]
            tunnel: w564 -> [_ _ _ _ _ _ _ _ w617 _ _ _]
            tunnel: w562 -> [_ _ _ _ _ _ _ _ _ w622 _ _]
            tunnel: w561 -> [_ _ _ _ _ _ _ _ _ _ w627 _]
            tunnel: w560 -> [_ _ _ _ _ _ _ _ _ _ _ w632]
            frame #0 {
              n203 = Unbundle By Name(w579) -> ("系数x"=w578:sgl)
              n204 = Concatenate Strings(w574, "x") -> (w573:string)
              n205 = call-poly <vilib>:"Write Key.vi"("section"=w576, "value"=w578, "key"=w573, "refnum"=w577) -> ()  [unwired: 5 in, 3 out]
            }
            frame #1 {
              n206 = Unbundle By Name(w586) -> ("系数+"=w585:sgl)
              n207 = Concatenate Strings(w581, "+") -> (w580:string)
              n208 = call-poly <vilib>:"Write Key.vi"("section"=w583, "value"=w585, "key"=w580, "refnum"=w584) -> ()  [unwired: 5 in, 3 out]
            }
            frame #2 {
              n209 = Unbundle By Name(w591) -> ("上限"=w590:sgl)
              n210 = call-poly <vilib>:"Write Key.vi"("section"=w587, "value"=w590, "key"=w588, "refnum"=w589) -> ()  [unwired: 5 in, 3 out]
            }
            frame #3 {
              n211 = Unbundle By Name(w596) -> ("下限"=w595:sgl)
              n212 = call-poly <vilib>:"Write Key.vi"("section"=w592, "value"=w595, "key"=w593, "refnum"=w594) -> ()  [unwired: 5 in, 3 out]
            }
            frame #4 {
              n213 = Unbundle By Name(w601) -> ("Ymax"=w600:dbl)
              n214 = call-poly <vilib>:"Write Key.vi"("section"=w597, "value"=w600, "key"=w598, "refnum"=w599) -> ()  [unwired: 5 in, 3 out]
            }
            frame #5 {
              n215 = Unbundle By Name(w606) -> ("Ymin"=w605:dbl)
              n216 = call-poly <vilib>:"Write Key.vi"("section"=w602, "value"=w605, "key"=w603, "refnum"=w604) -> ()  [unwired: 5 in, 3 out]
            }
            frame #6 {
              n217 = Unbundle By Name(w611) -> ("点数"=w610:dbl)
              n218 = call-poly <vilib>:"Write Key.vi"("section"=w607, "value"=w610, "key"=w608, "refnum"=w609) -> ()  [unwired: 5 in, 3 out]
            }
            frame #7 {
              n219 = Unbundle By Name(w616) -> ("起点"=w615:dbl)
              n220 = call-poly <vilib>:"Write Key.vi"("section"=w612, "value"=w615, "key"=w613, "refnum"=w614) -> ()  [unwired: 5 in, 3 out]
            }
            frame #8 {
              n221 = Unbundle By Name(w621) -> ("终点"=w620:dbl)
              n222 = call-poly <vilib>:"Write Key.vi"("section"=w617, "value"=w620, "key"=w618, "refnum"=w619) -> ()  [unwired: 5 in, 3 out]
            }
            frame #9 {
              n223 = Unbundle By Name(w626) -> ("上参考"=w625:sgl)
              n224 = call-poly <vilib>:"Write Key.vi"("section"=w622, "value"=w625, "key"=w623, "refnum"=w624) -> ()  [unwired: 5 in, 3 out]
            }
            frame #10 {
              n225 = Unbundle By Name(w631) -> ("下参考"=w630:sgl)
              n226 = call-poly <vilib>:"Write Key.vi"("section"=w627, "value"=w630, "key"=w628, "refnum"=w629) -> ()  [unwired: 5 in, 3 out]
            }
            frame #11 {
              n227 = Unbundle By Name(w636) -> ("基准"=w635:sgl)
              n228 = call-poly <vilib>:"Write Key.vi"("section"=w632, "value"=w635, "key"=w633, "refnum"=w634) -> ()  [unwired: 5 in, 3 out]
            }
          }
        }
        frame #6 {
          n229 = call <vilib>:"Close Config Data.vi"("refnum"=w637) -> ()  [unwired: 9 in, 2 out]
        }
      }
    }
    frame Error {
      n230 = call <vilib>:"Close Config Data.vi"("write file if changed (T)"=FALSE, "refnum"=w639) -> ()  [unwired: 8 in, 2 out]
    }
  }
